vi "SUM_CONTROLLLED_CONTROL.vi"(0 "connection ID in":refnum<k5>, 1 "Channel Enable":i32(slide) scale=0.0..6.0, 2 "Attenuation Select":i32(slide) scale=0.0..15.0, 3 "Clipping Select":i32(slide)=1 scale=1.0..3.0, 4 "Ib Clip select":i32(slide)=63 scale=0.0..63.0, 5 "error in":errorcluster) -> (14 "connection ID out":refnum<k5>, 19 "error out":errorcluster)   [LabVIEW 2012]
panel:
  in  "Sum/Maj":bool=TRUE
  in  "Delay Enable":i32(slide) scale=0.0..31.0
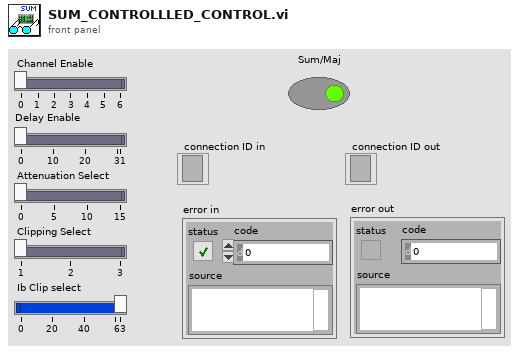
[diagram p1: front panel]
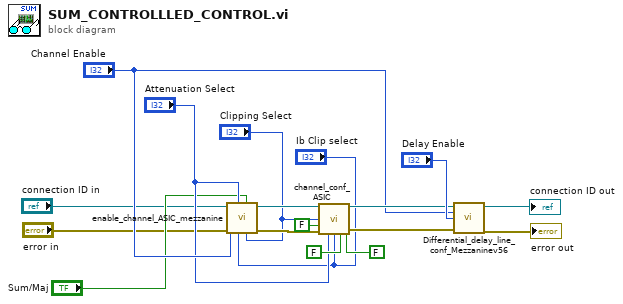
[diagram p0: block diagram]
diagram:
  n1 = call "enable_channel_ASIC_mezzanine.vi"("Clip_sel_b"="Clipping Select", "maj/sum"="Sum/Maj", "Ib_clipVb"="Ib Clip select", "Att gain"="Attenuation Select", "error in"="error in", "Channel"="Channel Enable", "connection ID"="connection ID in") -> ("error out"=w14:errorcluster, "connection ID out"=w13:refnum<k5>)  [unwired: 2 in, 1 out]
  n2 = call "channel_conf_ASIC.vi"("connection ID"=w13, "Clip_sel_b"="Clipping Select", "CompBuf_en_b"=FALSE, "error out"=w14, "Att gain"="Attenuation Select", "Ib_ClipVb"="Ib Clip select", "Clip_en_b"=FALSE, "Att_en_b"=FALSE) -> ("connection ID out"=w8:refnum<k5>, "error out 2"=w9:errorcluster)  [unwired: 3 in, 3 out]
  n3 = call "Differential_delay_line_conf_Mezzaninev56.vi"("connection ID"=w8, "channel"="Channel Enable", "Delay value"="Delay Enable", "error in (no error)"=w9) -> ("connection ID out"=→"connection ID out":refnum<k5>, "error out 2"=→"error out":errorcluster)  [unwired: 4 in, 6 out]
